vi "init_OSC.vi"(8 "error in (no error)":errorcluster, 10 "reset (f)":bool, 11 "VISA resource name":refnum<visa-resource-name>) -> (0 "error out":errorcluster, 3 "VISA resource name out":refnum<visa-resource-name>)   [LabVIEW 2012]
doc: "Establishes communication with the instrument and performs an instrument reset. \n\nThis VI also places the instrument in a default state needed for other instrument driver operations."
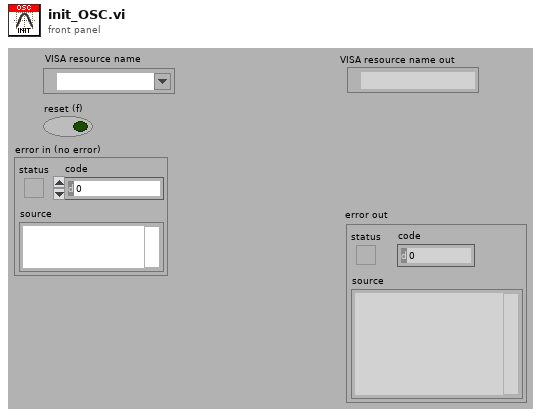
[diagram p1: front panel]
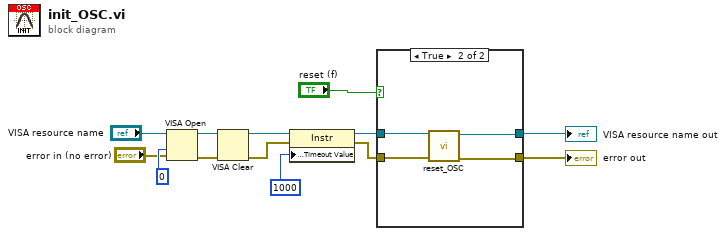
[diagram p0: block diagram]
diagram:
  n1 = VISA Open(access mode=u32 0, error in (no error)="error in (no error)", VISA resource name="VISA resource name") -> (VISA resource name=w11:refnum<visa-resource-name>, error out=w10:errorcluster)  [unwired: 2 in]
  n2 = VISA Clear(VISA resource name=w11, error in (no error)=w10) -> (VISA resource name out=w9:refnum<visa-resource-name>, error out=w8:errorcluster)
  n3 = property on="Property Node" class="Instr"(reference=w9, error in=w8, "General Settings:Timeout Value"=u32 1000) -> (reference out=w6:refnum<visa-resource-name>, error out=w5:errorcluster)
  n4 = case shown="True" "reset (f)" {
    tunnel: [w14 w17] -> w2
    tunnel: [w15 w16] -> w1
    tunnel: w6 -> [w14 w19]
    tunnel: w5 -> [w15 w18]
    frame False {
    }
    frame True {
      n5 = call "reset_OSC.vi"("error in (no error)"=w18, "VISA resource name"=w19) -> ("error out"=w16:errorcluster, "VISA resource name out"=w17:refnum<visa-resource-name>)  [unwired: 8 in]
    }
  }
  "VISA resource name out" <- w2
  "error out" <- w1
